vi "GetAttributes.vi"(0 "MLA":refnum<class "MLA.lvclass">, 1 "OnlyGetDvrReference(False)":bool, 5 "error in (no error)":errorcluster) -> (14 "MLA":refnum<class "MLA.lvclass">, 15 "Data":T1={"App Name"="", "App Version"="", "Revision History"="", "Log File Path"=path "C:/Projects/seneca5_korrykdm340/Data", "Config INI File"=path "C:/Projects/seneca5_korrykdm340/Data", "Config Path"=path "C:/Projects/seneca5_korrykdm340/Data", "Log Archive Path"=path "C:/Projects/seneca5_korrykdm340/Data", "Msg Q's"=[], "VI"=refnum, "ErrLog"=refnum}, 17 "DataRef":refnum<data-value>, 19 "error out":errorcluster)   [LabVIEW 2017, in "MLA.lvclass"]
uses:
  MLA.lvclass
  protected/ObjectAttributes.ctl
  S5Tools/ErrorLog/ErrorLog.lvclass
  MLA.lvclass/MLA.ctl
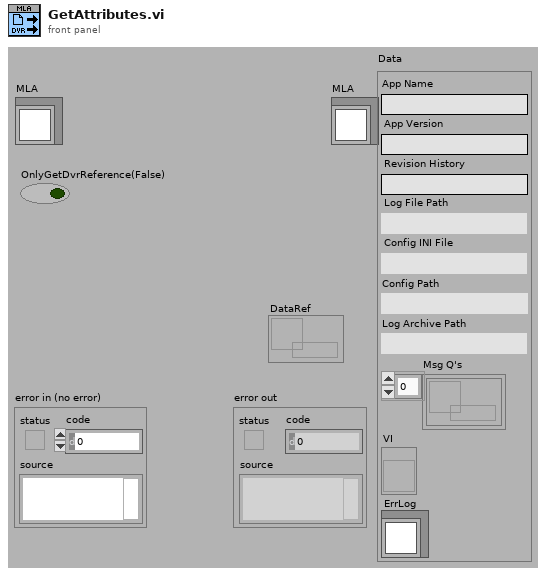
[diagram p1: front panel]
types:
  T1 = typedef "MLA.lvclass/ObjectAttributes.ctl" = cluster{"App Name":string, "App Version":string, "Revision History":string, "Log File Path":path, "Config INI File":path, "Config Path":path, "Log Archive Path":path, "Msg Q's":refnum<queue>[], "VI":refnum<vi>, "ErrLog":refnum<class "ErrorLog.lvclass">}
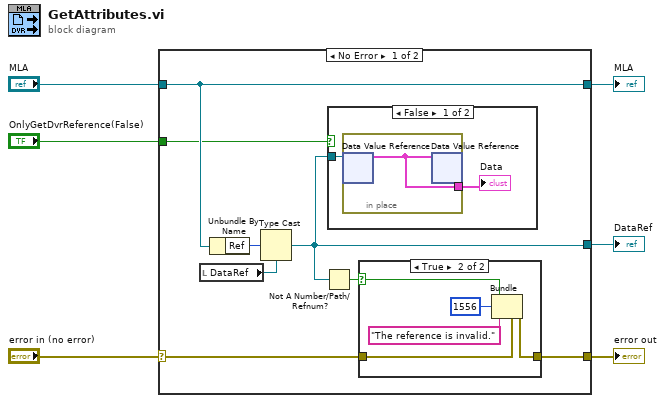
[diagram p0: block diagram]
diagram:
  n1 = case shown="No Error" "error in (no error)" {
    selector: "error in (no error)" -> [w10 w24]
    tunnel: [w7 w24] -> w5
    tunnel: [w14 w25] -> w3
    tunnel: "MLA" -> [w14 w25]
    tunnel: [w8 _] -> w2
    tunnel: "OnlyGetDvrReference(False)" -> [w11 _]
    frame No Error {
      n2 = local read "DataRef"() -> (w12:refnum<data-value>)
      n3 = Unbundle By Name(w14) -> ("Ref"=w13:u32)
      n4 = Type Cast(type=w12, x=w13) -> (*(type *) &x=w8:refnum<data-value>)
      n5 = Not A Number/Path/Refnum?(number/path/refnum=w8) -> (NaN/Path/Refnum?=w9:bool)
      n6 = case shown="False" w11 {
        tunnel: w8 -> [w22 _]
        frame False {
          n7 = in-place {
            in-place-border: [w23] -> w21
            n8 = in-place-dvr #1(w22) -> (w23:T1)  [unwired: 1 out]
            n9 = in-place-dvr #1(w23) -> ()  [unwired: 2 out]
          }
          "Data" <- w21
        }
        frame True {
        }
      }
      n10 = case shown="True" w9 {
        selector: w9 -> [_ w18]
        tunnel: w10 -> [w15 w20]
        tunnel: [w15 w19] -> w7
        frame False {
        }
        frame True {
          n11 = Bundle(cluster=w20, "status"=w18, "code"=1556, "source"="The reference is invalid.") -> (w19:errorcluster)
        }
      }
    }
    frame Error {
    }
  }
  "error out" <- w5
  "MLA" <- w3
  "DataRef" <- w2
